vi "terminateLidar.vi"(3 "error in":errorcluster, 5 "VISA resource name":refnum<visa-resource-name>) -> (0 "stop":bool)   [LabVIEW 2016]
uses:
  <instrlib>/Hokuyo URG Series/Hokuyo URG Series.lvlib
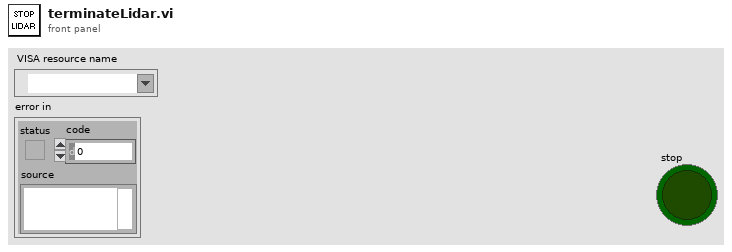
[diagram p1: front panel]
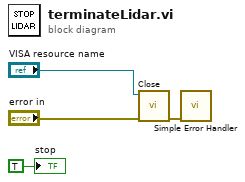
[diagram p0: block diagram]
diagram:
  n1 = call <instrlib>:"Close.vi"("error in (no error)"="error in", "VISA resource name"="VISA resource name") -> ("error out"=w4:errorcluster)  [unwired: 9 in]
  n2 = call <vilib>:"Simple Error Handler.vi"("error in (no error)"=w4) -> ()  [unwired: 4 in, 5 out]
  "stop" <- TRUE ("stop")
